vi "_error_gen.vi"(11 "return type":i32) -> (0 "error out":errorcluster)   [LabVIEW 2019, in "UV-VIS_AVANTES.lvclass"]
uses:
  UV-VIS_AVANTES.lvclass
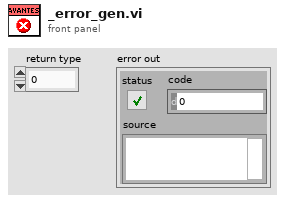
[diagram p1: front panel]
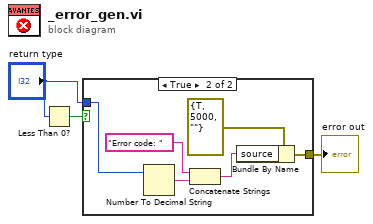
[diagram p0: block diagram]
diagram:
  n1 = Less Than 0?(x="return type") -> (x < 0?=w1:bool)
  n2 = case shown="True" w1 {
    tunnel: "return type" -> [_ w8]
    tunnel: [_ w4] -> w3
    frame False {
    }
    frame True {
      n3 = Number To Decimal String(number=w8) -> (decimal integer string=w7:string)  [unwired: 1 in]
      n4 = Concatenate Strings("Error code: ", w7) -> (w5:string)
      n5 = Bundle By Name(cluster=errorcluster {"status"=TRUE, "code"=5000, "source"=""} ("error constant"), "source"=w5) -> (w4:errorcluster)
    }
  }
  "error out" <- w3
